vi "RobotDriveOpen6MotorWithTalonSR.vi"(0 "Left Motor 1":T1=enum."Invalid", 1 "Left Motor 2":T1=enum."Invalid", 2 "Left Motor 3":T1=enum."Invalid", 3 "Right Motor 1":T1=enum."Invalid", 4 "Right Motor 2":T1=enum."Invalid", 5 "Right Motor 3":T1=enum."Invalid", 7 "error in (no error)":errorcluster, 8 "Left Motor 1 Inverted":bool, 9 "Right Motor 1 Inverted":bool, 10 "Left Motor 2 Inverted":bool, 11 "Right Motor 2 Inverted":bool, 12 "Left Motor 3 Inverted":bool, 13 "Right Motor 3 Inverted":bool) -> (20 "RobotDriveDevRef":T2={"DevStatus"={"status"=FALSE, "code"=0, "source"=""}, "Motors[]"=[], "Square Inputs"=FALSE, "Max Output"=1.0}, 27 "error out":errorcluster)   [LabVIEW 2016, in "ArgosLib.lvlib"]
doc: "Opens a reference to the robot drive for a two-, four-, or six-motor robot using Talon SR motor controllers connected via PWM.\n\nFor 2-motor drive, connect Left Motor 1 and Right Motor 1.\nFor 4-motor drive, connect Left Motor 2 and Right Motor 2 in addition to the 2-motor drive connections.\nFor 6-motor drive, connect Left Motor 3 and Right Motor 3 in addition to the 4-motor drive connections.\n\nInversions are optional and are set to false if disconnected.\n\nThis software is licensed. Open the labview\\readme\\WPI Robotics Library Open Source License.txt file for more information."
uses:
  <vilib>/Rock Robotics/WPI/RobotDrive/WPI_RobotDriveDevRef.ctl
  <vilib>/Rock Robotics/WPI/MotorControl/WPI_MotorControlDeviceRef.ctl
  <vilib>/Rock Robotics/WPI/MotorControl/WPI_MotorControlType.ctl
  <vilib>/Rock Robotics/SystemInterfaces/DIO/FPGA_DIOPWMChannel.ctl
  <vilib>/Rock Robotics/WPI/PWM/WPI_PWMDeadband.ctl
  <vilib>/Rock Robotics/WPI/SafetyOutput/WPI_SafetyOutputConfigMenu.ctl
  <vilib>/Rock Robotics/WPI/MotorControl/WPI_MotorControlOpen Talon.vi
  ArgosLib.lvlib
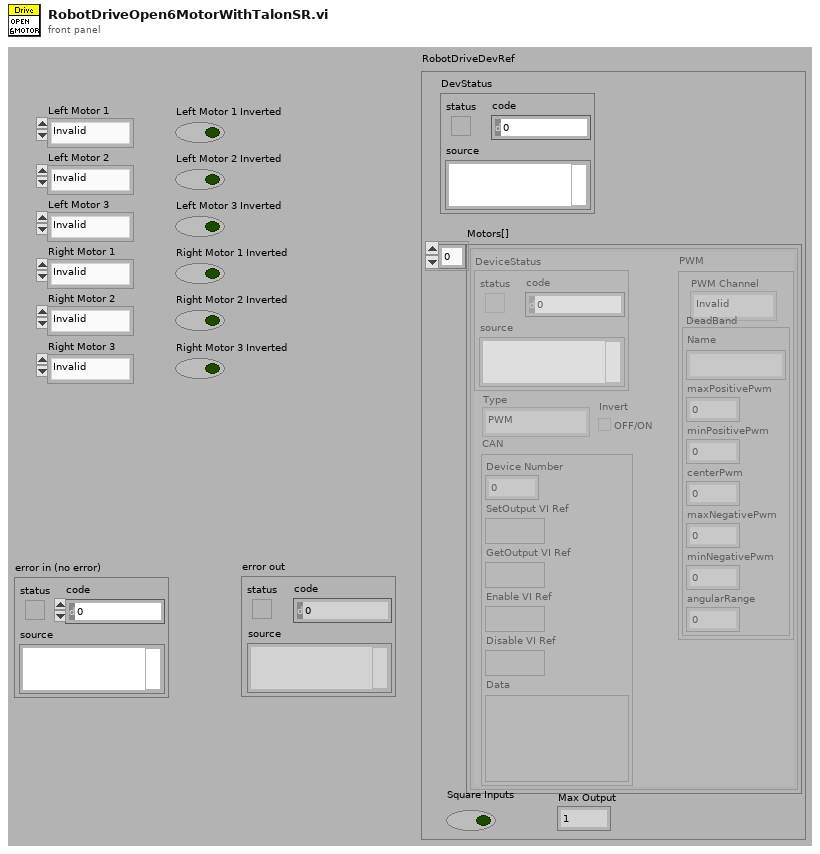
[diagram p1: front panel]
types:
  T1 = typedef "FPGA_DIOPWMChannel.ctl" = enum8{"PWM 0", "PWM 1", "PWM 2", "PWM 3", "PWM 4", "PWM 5", "PWM 6", "PWM 7", "PWM 8", "PWM 9", "PWM MXP 0", "PWM MXP 1", "PWM MXP 2", "PWM MXP 3", "PWM MXP 4", "PWM MXP 5", "PWM MXP 6", "PWM MXP 7", "PWM MXP 8", "PWM MXP 9", "Invalid"}
  T2 = typedef "WPI_RobotDriveDevRef.ctl" = cluster{"DevStatus":errorcluster, "Motors[]":T3[], "Square Inputs":bool, "Max Output":dbl}
  T3 = typedef "WPI_MotorControlDeviceRef.ctl" = cluster{"DeviceStatus":errorcluster, "Type":T4, "PWM":cluster{"PWM Channel":T1, "DeadBand":T5}, "CAN":cluster{"Device Number":u8, "SetOutput VI Ref":variant, "GetOutput VI Ref":variant, "Enable VI Ref":variant, "Disable VI Ref":variant, "Data":variant}, "Invert":bool}
  T4 = typedef "WPI_MotorControlType.ctl" = enum16{"PWM", "CAN"}
  T5 = typedef "WPI_PWMDeadband.ctl" = cluster{"Name":string, "maxPositivePwm":i32, "minPositivePwm":i32, "centerPwm":i32, "maxNegativePwm":i32, "minNegativePwm":i32, "angularRange":u16}
  T6 = typedef "WPI_SafetyOutputConfigMenu.ctl" = enum16{"Enable", "Disable"}
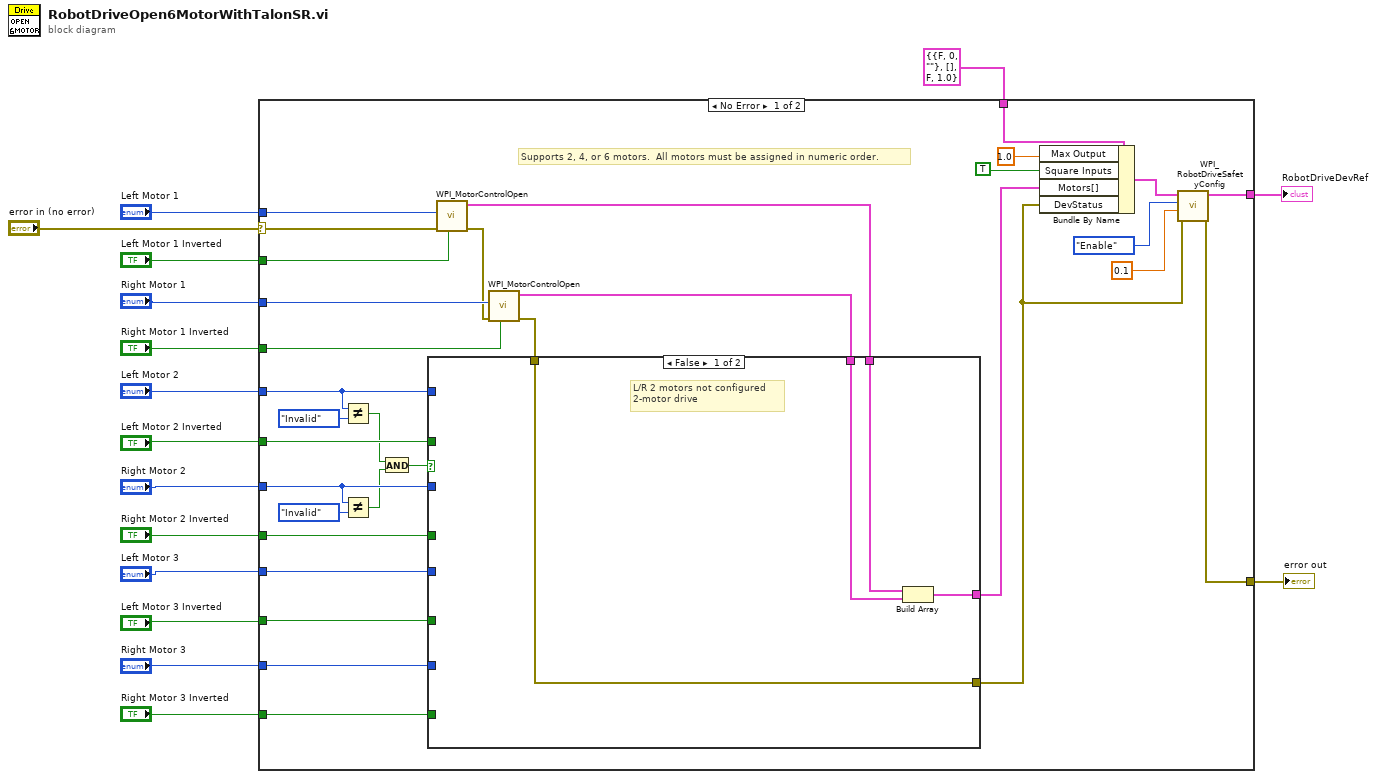
[diagram p0: block diagram]
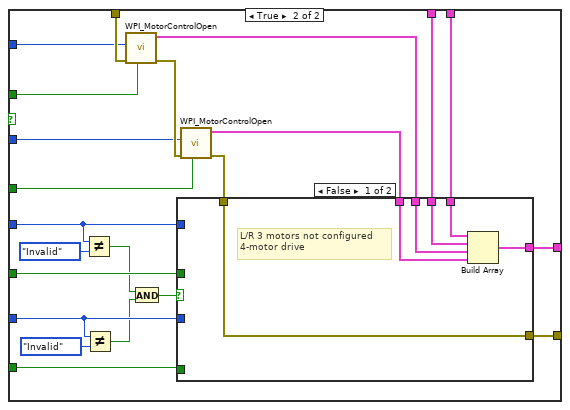
[diagram p2: hidden frame]
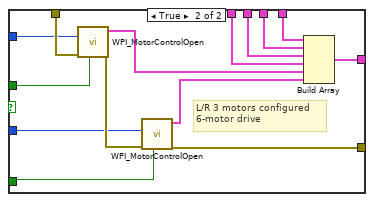
[diagram p3: hidden frame]
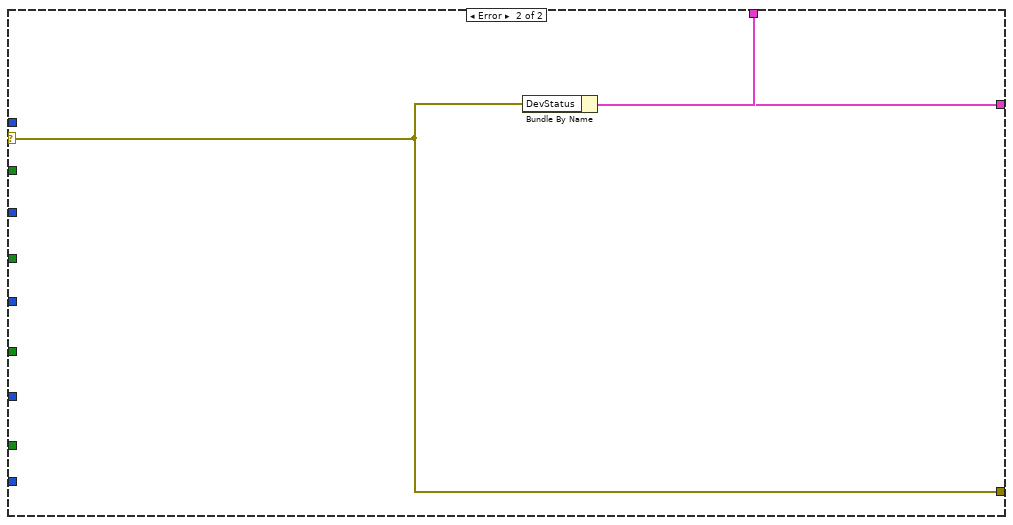
[diagram p4: hidden frame]
diagram:
  n1 = case shown="No Error" "error in (no error)" {
    selector: "error in (no error)" -> [w17 w95]
    tunnel: [w36 w96] -> w16
    tunnel: T2 {"DevStatus"={"status"=FALSE, "code"=0, "source"=""}, "Motors[]"=[], "Square Inputs"=FALSE, "Max Output"=1.0} ("RobotDriveDevRef") -> [w48 w97]
    tunnel: "Right Motor 2" -> [w24 _]
    tunnel: "Left Motor 2" -> [w27 _]
    tunnel: "Right Motor 1" -> [w46 _]
    tunnel: "Left Motor 1 Inverted" -> [w43 _]
    tunnel: "Right Motor 1 Inverted" -> [w42 _]
    tunnel: "Right Motor 2 Inverted" -> [w40 _]
    tunnel: "Left Motor 2 Inverted" -> [w41 _]
    tunnel: [w37 w95] -> w9
    tunnel: "Left Motor 3" -> [w33 _]
    tunnel: "Left Motor 3 Inverted" -> [w31 _]
    tunnel: "Right Motor 3" -> [w32 _]
    tunnel: "Right Motor 3 Inverted" -> [w30 _]
    tunnel: "Left Motor 1" -> [w28 _]
    frame No Error {
      # "Supports 2, 4, or 6 motors.  All motors must be assigned in numeric order."
      n2 = Not Equal?(x=w27, y=FPGA_DIOPWMChannel."Invalid") -> (x != y?=w23:bool)
      n3 = Not Equal?(x=w24, y=FPGA_DIOPWMChannel."Invalid") -> (x != y?=w22:bool)
      n4 = And(x=w23, y=w22) -> (x .and. y?=w21:bool)
      n5 = call-poly <vilib>:"WPI_MotorControlOpen.vi"("Invert"=w43, "error in (no error)"=w17, "PWM Channel"=w28) -> ("error out"=w44:errorcluster, "MotorControlDeviceRef"=w18:T3)  [unwired: 1 in, 6 out]
      n6 = call-poly <vilib>:"WPI_MotorControlOpen.vi"("Invert"=w42, "error in (no error)"=w44, "PWM Channel"=w46) -> ("error out"=w45:errorcluster, "MotorControlDeviceRef"=w19:T3)  [unwired: 1 in, 6 out]
      n7 = case shown="False" w21 {
        tunnel: w45 -> [w52 w73]
        tunnel: w41 -> [_ w72]
        tunnel: w40 -> [_ w71]
        tunnel: w33 -> [_ w62]
        tunnel: w32 -> [_ w61]
        tunnel: w31 -> [_ w69]
        tunnel: w30 -> [_ w68]
        tunnel: [w52 w67] -> w29
        tunnel: w27 -> [_ w66]
        tunnel: w24 -> [_ w65]
        tunnel: [w49 w57] -> w20
        tunnel: w19 -> [w50 w54]
        tunnel: w18 -> [w51 w53]
        frame False {
          # "L/R 2 motors not configured\n2-motor drive"
          n8 = Build Array(w51, w50) -> (w49:T3[])
        }
        frame True {
          n9 = Not Equal?(x=w62, y=FPGA_DIOPWMChannel."Invalid") -> (x != y?=w60:bool)
          n10 = Not Equal?(x=w61, y=FPGA_DIOPWMChannel."Invalid") -> (x != y?=w59:bool)
          n11 = call-poly <vilib>:"WPI_MotorControlOpen.vi"("Invert"=w72, "error in (no error)"=w73, "PWM Channel"=w66) -> ("error out"=w74:errorcluster, "MotorControlDeviceRef"=w55:T3)  [unwired: 1 in, 6 out]
          n12 = And(x=w60, y=w59) -> (x .and. y?=w58:bool)
          n13 = call-poly <vilib>:"WPI_MotorControlOpen.vi"("Invert"=w71, "error in (no error)"=w74, "PWM Channel"=w65) -> ("error out"=w70:errorcluster, "MotorControlDeviceRef"=w56:T3)  [unwired: 1 in, 6 out]
          n14 = case shown="False" w58 {
            tunnel: w70 -> [w80 w94]
            tunnel: w69 -> [_ w92]
            tunnel: w68 -> [_ w91]
            tunnel: [w80 w90] -> w67
            tunnel: w62 -> [_ w89]
            tunnel: w61 -> [_ w88]
            tunnel: [w79 w87] -> w57
            tunnel: w56 -> [w75 w84]
            tunnel: w55 -> [w76 w83]
            tunnel: w54 -> [w77 w82]
            tunnel: w53 -> [w78 w81]
            frame False {
              # "L/R 3 motors not configured\n4-motor drive"
              n15 = Build Array(w78, w77, w76, w75) -> (w79:T3[])
            }
            frame True {
              # "L/R 3 motors configured\n6-motor drive"
              n16 = call-poly <vilib>:"WPI_MotorControlOpen.vi"("Invert"=w92, "error in (no error)"=w94, "PWM Channel"=w89) -> ("error out"=w93:errorcluster, "MotorControlDeviceRef"=w85:T3)  [unwired: 1 in, 6 out]
              n17 = call-poly <vilib>:"WPI_MotorControlOpen.vi"("Invert"=w91, "error in (no error)"=w93, "PWM Channel"=w88) -> ("error out"=w90:errorcluster, "MotorControlDeviceRef"=w86:T3)  [unwired: 1 in, 6 out]
              n18 = Build Array(w81, w82, w83, w84, w85, w86) -> (w87:T3[])
            }
          }
        }
      }
      n19 = Bundle By Name(cluster=w48, "Max Output"=1.0, "Square Inputs"=TRUE ("DestroyPWM?"), "Motors[]"=w20, "DevStatus"=w29) -> (w38:T2)
      n20 = call <vilib>:"WPI_RobotDriveSafetyConfig.vi"("error in (no error)"=w29, "timeout (s)"=0.1, "mode"=WPI_SafetyOutputConfigMenu."Enable", "RobotDriveDevRef"=w38) -> ("error out"=w37:errorcluster, "RobotDriveDevRef"=w36:T2)  [unwired: 6 out]
    }
    frame Error {
      n21 = Bundle By Name(cluster=w97, "DevStatus"=w95) -> (w96:T2)
    }
  }
  "RobotDriveDevRef" <- w16
  "error out" <- w9
